vi "MAIN PS.vi"(11 "Elettrotest PS 2":refnum<vi>) -> ()   [LabVIEW 2019]
uses:
  TypeDef/ELATTROTEST PS.ctl
  TypeDef/DEVICE NAME.ctl
  <vilib>/Utility/file.llb/Read From Spreadsheet File (string).vi
  <vilib>/Instr/_visa.llb/VISA Configure Serial Port (Instr).vi
  Freq elettrotest PS global.vi
panel:
  out "error out 3":errorcluster
  out "# elements in queue":i32
  in  "Elettrotest PS":T1={"TENSIONE[V]"=230.0, "FREQ[Hz]"=50.0, "T rampa[s]"=5.0, "imposta"=FALSE, "V out [Hz]"=0.0, "F out [Hz]"=0.0, "ACK"=FALSE, "Remoto?"=FALSE, "ctrl remoto"=FALSE} {"FREQ[Hz]" min=45.0 max=65.0; "TENSIONE[V]" min=0.0 max=500.0}
  out "CK DATO":bool
  in  "remoto":bool
  in  "s":bool
  in  "SET RAMPE":bool
  in  "COMANDO":T2={"NU"=FALSE, "OUT"=FALSE, "REMOTO"=TRUE, "DC"=FALSE, "SINK"=FALSE, "MONO"=FALSE, "SENSE"=FALSE, "PORTATA"=TRUE}
  in  "rampa tensione frequenza all 2":T3
  out "Numeric":i32
  out "ACK":bool
  out "Timeout":bool
  out "Error Out":bool
  out "CK Tot":bool
  in  "EXIT":bool
  in  "Tab Control":enum32{"COM SETTINGS", "Page 2"}(tab)
  in  "baud rate (9600)":u32=1200
  in  "data bits (8)":u16=8 min=5 max=8 step=1
  in  "parity (0:none)":enum16{"None", "Odd", "Even", "Mark", "Space"}(ring)
  in  "timeout (10sec)":u32=10000
  in  "termination char\n(0xA = '\\n' = LF)":u8=10 format="%.0x"
  in  "stop bits (10: 1 bit)":u16(ring)=10 items=["1.0"=10, "1.5"=15, "2.0"=20]
  in  "Enable Termination\nChar (T)":bool=TRUE
  out "error out":errorcluster
  out "COM":string
  out "error out 2":errorcluster
  out "Fase R":T4 {"Freq" format="%#.2g"; "Vout" format="%#.1f"; "Vset" format="%#.1f"}
  out "Fase S":T4 {"Fase" format="%#.0f"; "Freq" format="%#.2g"; "Vout" format="%#.1f"; "Vset" format="%#.1f"}
  out "Fase T":T4 {"Fase" format="%#.1f"; "Freq" format="%#.2g"; "Vout" format="%#.1f"; "Vset" format="%#.1f"}
  out "Modo R":T5
  out "Modo S":T5
  out "Modo T":T5
  out "Allarme S":T6
  out "Allarme R":T6
  out "AllarmeT":T6
  in  "flow control (0:none)":u16(ring) items=["None", "XON/XOFF", "RTS/CTS", "XON/XOFF & RTS/CTS", "DTR/DSR", "XON/XOFF & DTR/DSR"]
  out "STATO":string
  in  "rampa tensione frequenza":T7 {"tiporampa" items=["Tensione"=0, "Frequenza"=1, "Fase"=3]}
  in  "rampa tensione frequenza all":T3
  # "COMANDO T\\F"
  # "INVIA COMANDO"
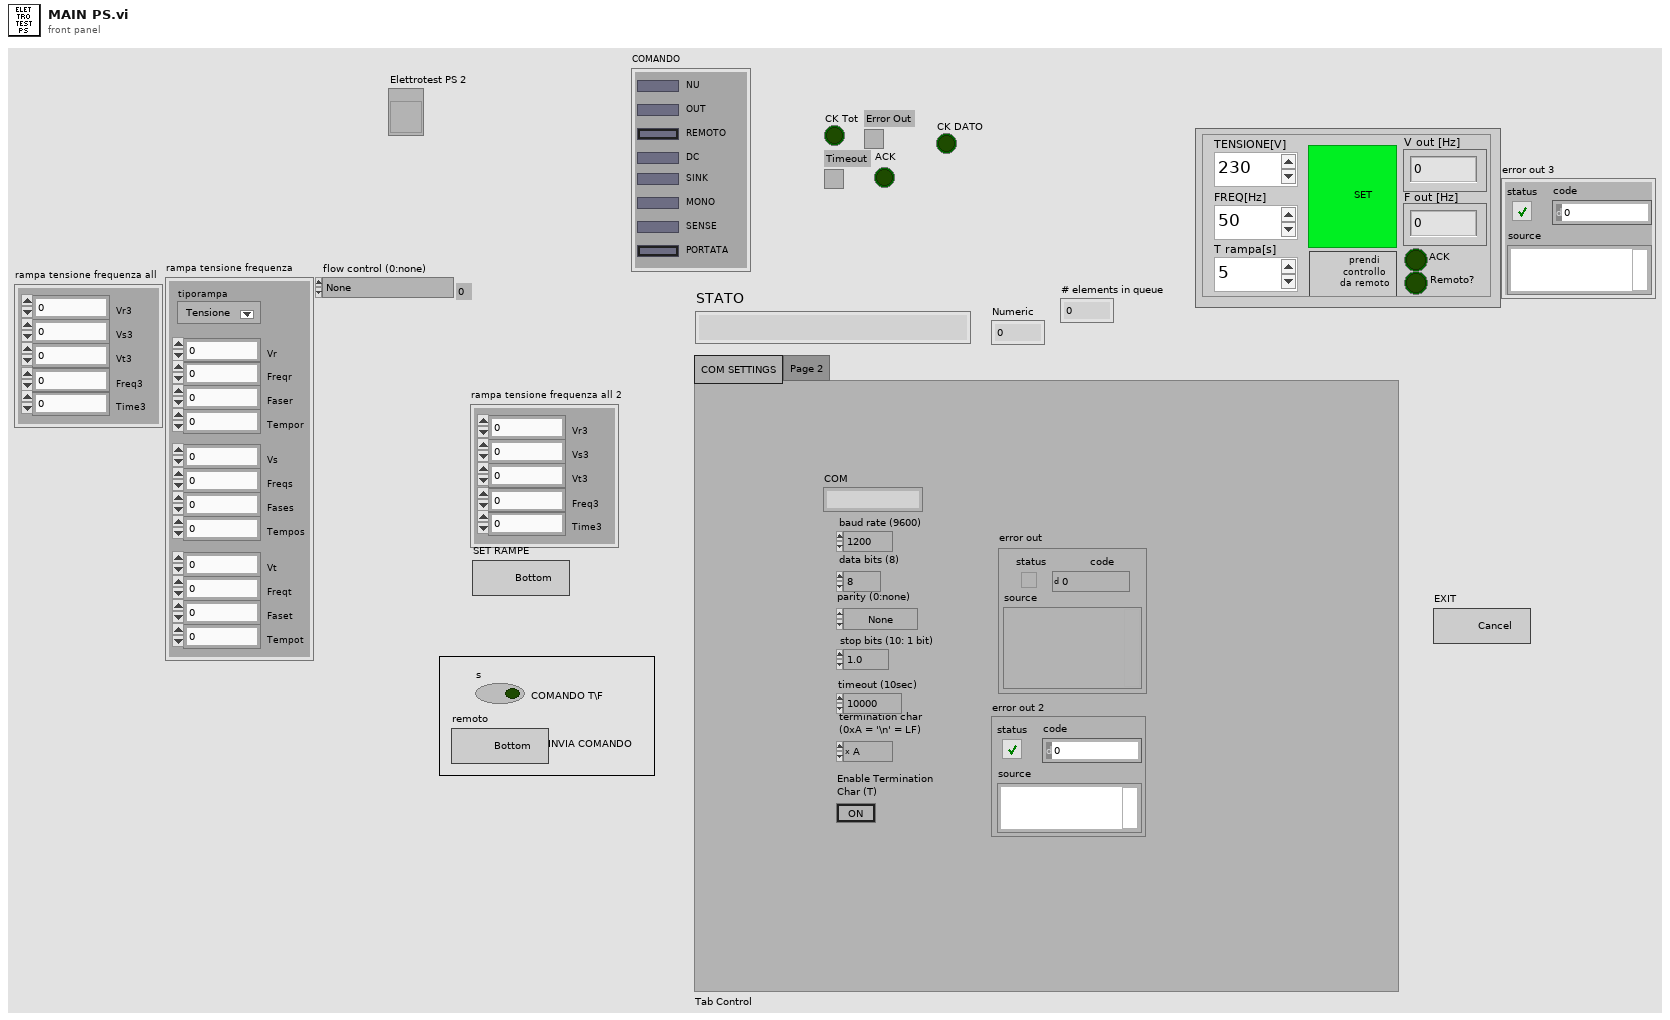
[diagram p1: front panel]
types:
  T1 = typedef "ELATTROTEST PS.ctl" = cluster{"TENSIONE[V]":dbl, "FREQ[Hz]":dbl, "T rampa[s]":dbl, "imposta":bool, "V out [Hz]":dbl, "F out [Hz]":dbl, "ACK":bool, "Remoto?":bool, "ctrl remoto":bool}
  T2 = cluster{"NU":bool, "OUT":bool, "REMOTO":bool, "DC":bool, "SINK":bool, "MONO":bool, "SENSE":bool, "PORTATA":bool}
  T3 = cluster{"Vr3":dbl, "Vs3":dbl, "Vt3":dbl, "Freq3":dbl, "Time3":dbl}
  T4 = cluster{"Vset":dbl, "Vout":dbl, "Iout":dbl, "Freq":dbl, "Fase":dbl, "Modo":dbl, "Allarmi":dbl}
  T5 = cluster{"Remote":bool, "3 Phase":bool, "DC":bool, "Portata alta":bool, "Out abilitata":bool, "Inrush abilitato":bool, "Sincronismo interno":bool, "4 Fili":bool}
  T6 = cluster{"Overvoltage":bool, "Undervoltage":bool, "Overtemperature":bool, "Inverter":bool, "Not used":bool, "DeltaV":bool, "Current limitation":bool, "Not used":bool}
  T7 = cluster{"Vr":dbl, "Tempor":dbl, "Freqr":dbl, "Faser":dbl, "Vs":dbl, "Freqs":dbl, "Fases":dbl, "Tempos":dbl, "Vt":dbl, "Freqt":dbl, "Faset":dbl, "Tempot":dbl, "tiporampa":u8}
  T8 = typedef "DEVICE NAME.ctl" = enum16{"WATTMETRO", "APLUS", "PLC BANCO 1", "PLC RACK", "PLC BANCO 2", "PS", "NI cDAQ", "RESISTOMAT"}
  T9 = enum16{"ALIGN -CENTER", "ALIGN -TOP LEFT", "ALIGN -AS IS", "ALIGN -CUSTOM"}
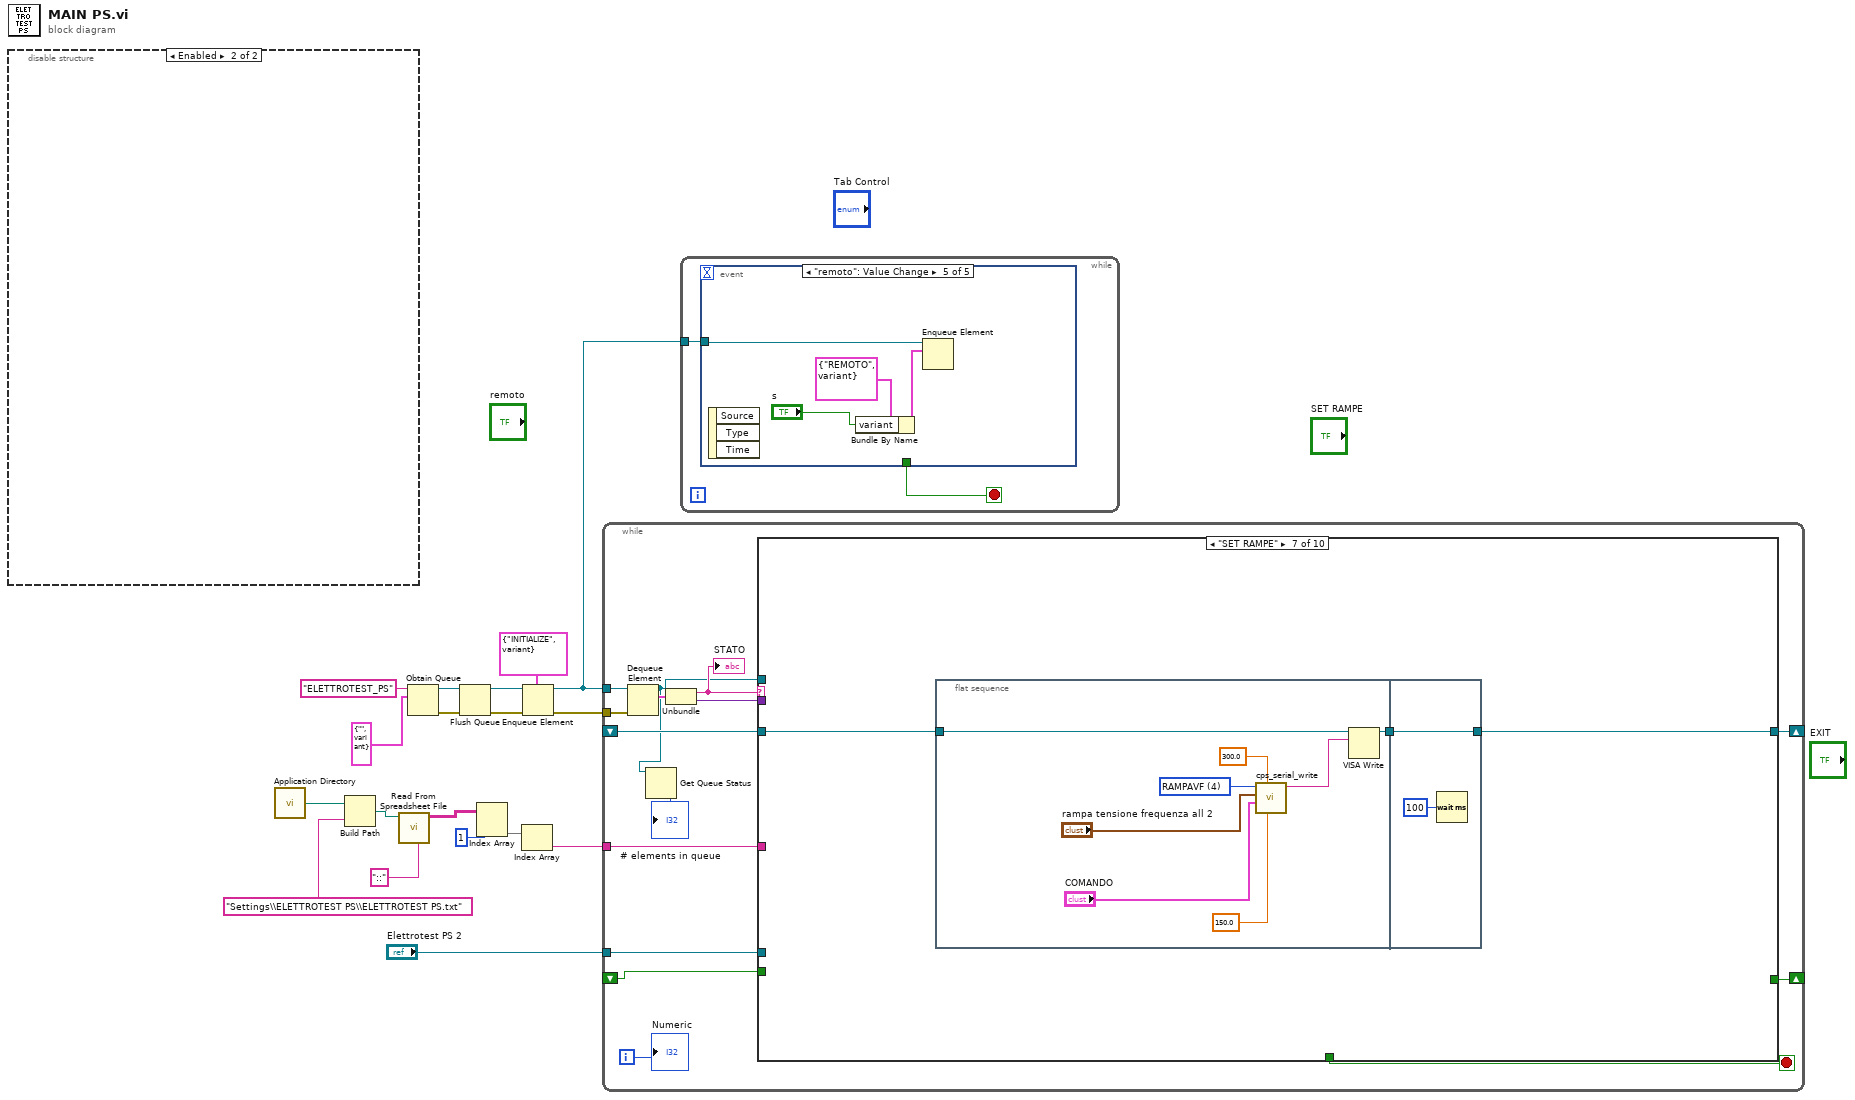
[diagram p0: block diagram]
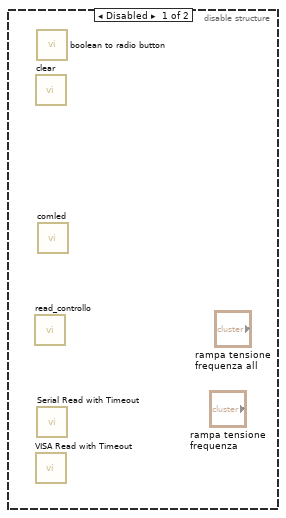
[diagram p2: hidden frame]
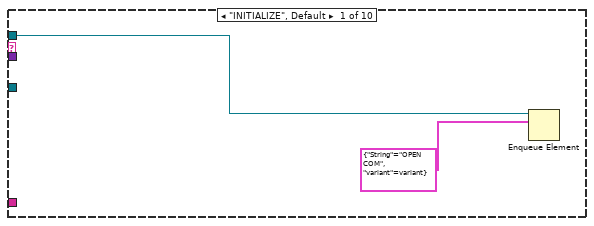
[diagram p3: hidden frame]
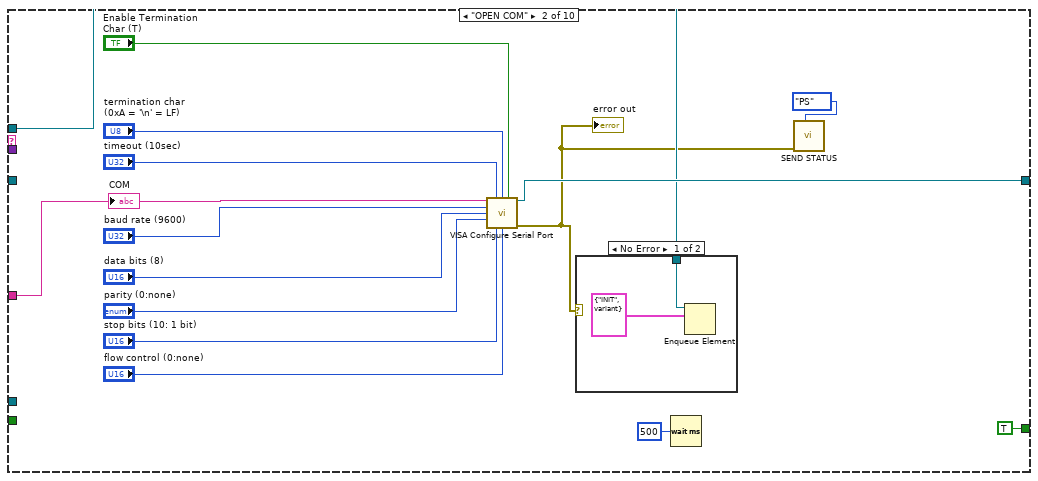
[diagram p4: hidden frame]
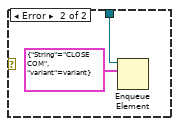
[diagram p5: hidden frame]
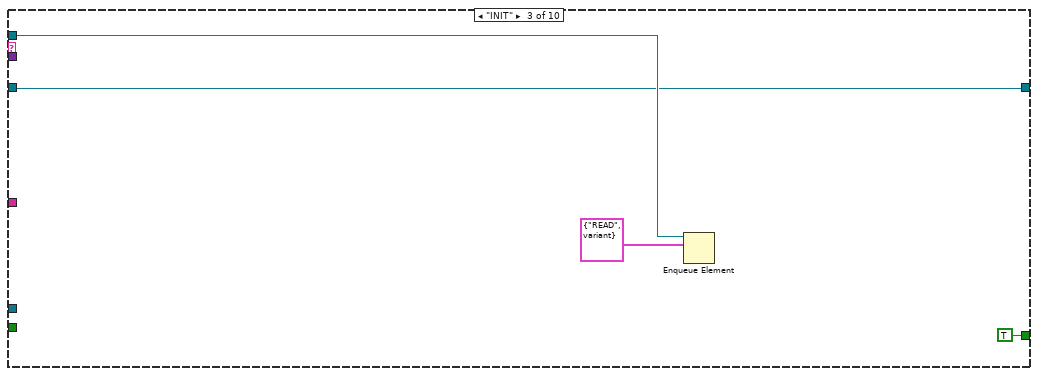
[diagram p6: hidden frame]
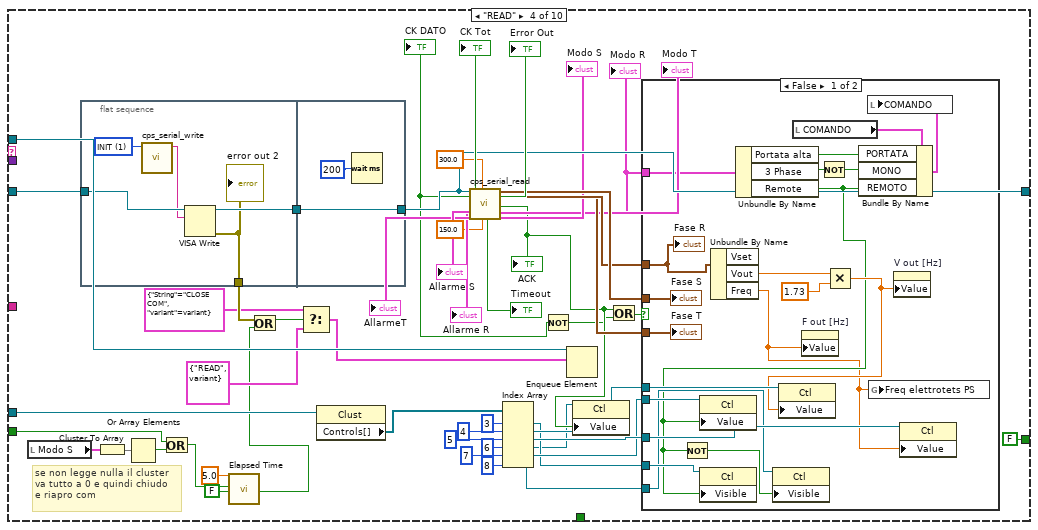
[diagram p7: hidden frame]
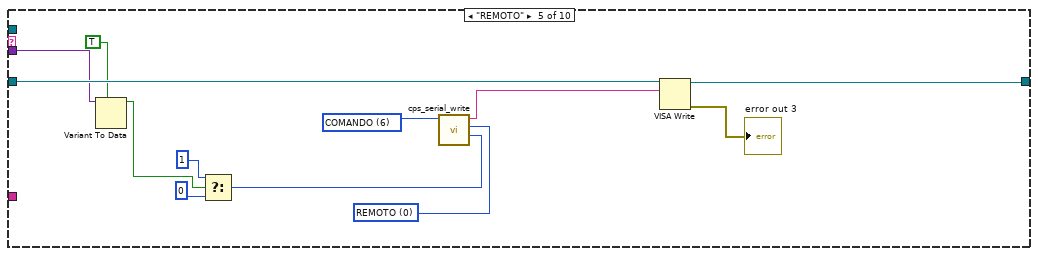
[diagram p9: hidden frame]
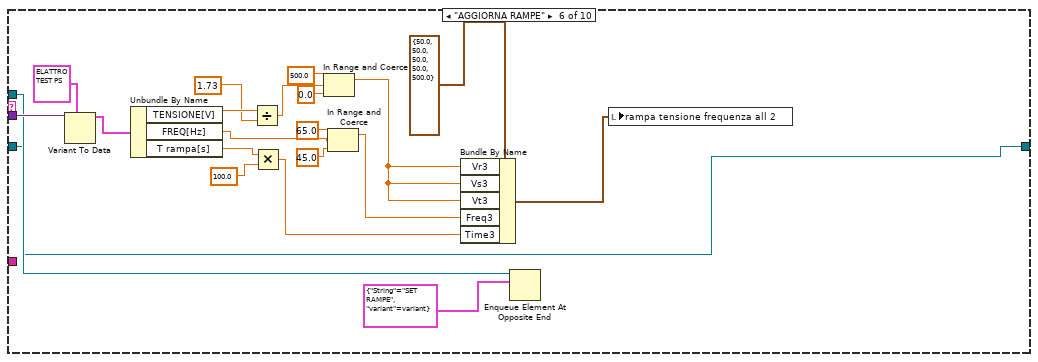
[diagram p10: hidden frame]
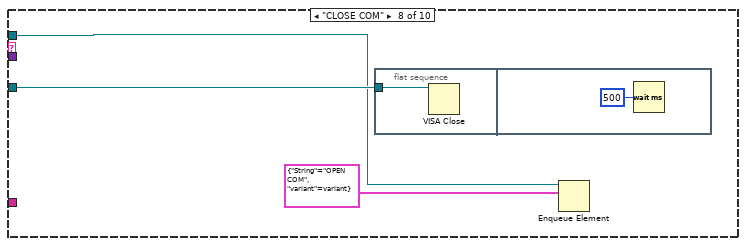
[diagram p11: hidden frame]
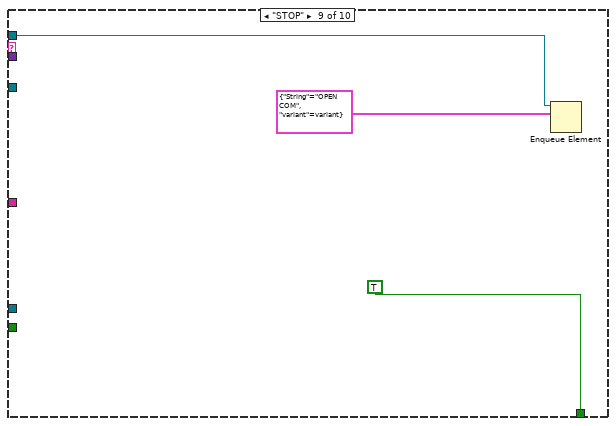
[diagram p12: hidden frame]
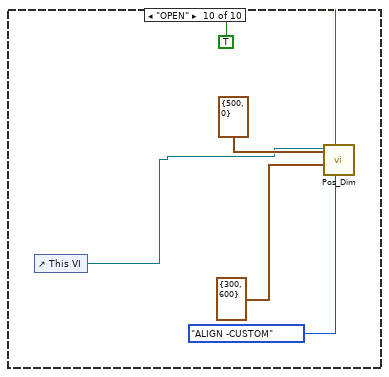
[diagram p13: hidden frame]
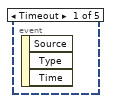
[diagram p14: hidden frame]
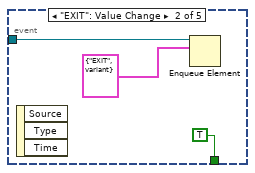
[diagram p15: hidden frame]
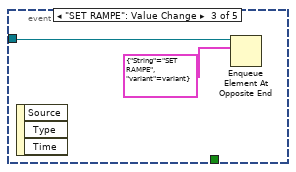
[diagram p16: hidden frame]
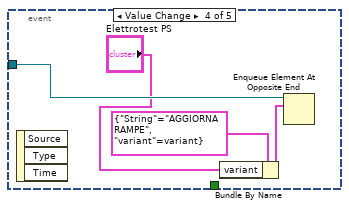
[diagram p17: hidden frame]
diagram:
  n1 = disable-structure shown="Enabled" {
    frame Disabled {
      n2 = call "read_controllo.vi"() -> ()  [unwired: 8 in, 1 out]
      n3 = call "clear.vi"() -> ()  [unwired: 1 in]
      n4 = call "VISA Read with Timeout.vi"() -> ()  [unwired: 4 in, 5 out]
      n5 = call "boolean to radio button.vi"() -> ()  [unwired: 1 in, 1 out]
      n6 = call "Serial Read with Timeout.vi"() -> ()  [unwired: 3 in, 3 out]
      n7 = call "comled.vi"() -> ()  [unwired: 1 in, 1 out]
    }
    frame Enabled {
    }
  }
  n8 = call <vilib>:"Application Directory.vi"() -> ("Application Directory"=w3:path)
  n9 = Build Path(base path=w3, name or relative path="Settings\\ELETTROTEST PS\\ELETTROTEST PS.txt") -> (appended path=w5:path)
  n10 = call-poly <vilib>:"Read From Spreadsheet File.vi"("delimiter (\\t)"="::" ("delimiter (\\t)"), "file path (dialog if empty)"=w5) -> ("all rows"=w7:string[][])  [unwired: 5 in, 4 out]
  n11 = Obtain Queue(name (unnamed)="ELETTROTEST_PS", element data type=cluster{"String":string, "variant":variant} {"String"="", "variant"=variant} ("element")) -> (queue out=w16:refnum<queue>, error out=w15:errorcluster)  [unwired: 3 in, 1 out]
  n12 = Flush Queue(queue=w16, error in (no error)=w15) -> (queue out=w14:refnum<queue>, error out=w13:errorcluster)  [unwired: 1 out]
  n13 = Index Array(array=w7, index (col)=1 ("disabled index (col)")) -> (element=w9:string[])  [unwired: 1 in]
  n14 = Index Array(array=w9) -> (element=w2:string)  [unwired: 1 in]
  n15 = Enqueue Element(queue=w14, element=cluster{"String":string, "variant":variant} {"String"="INITIALIZE", "variant"=variant}, error in (no error)=w13) -> (queue out=w10:refnum<queue>, error out=w12:errorcluster)  [unwired: 1 in, 1 out]
  n16 = while {
    tunnel: w10 -> [w33]
    tunnel: w12 -> [w32]
    shift-right: [w30] -> _
    shift-left: _ -> [w28]
    tunnel: w2 -> [w26]
    tunnel: "Elettrotest PS 2" -> [w25]
    shift-right: [w21] -> _
    shift-left: _ -> [w22]
    i -> [w27]
    stop <- w29 stop-if-true
    n17 = Dequeue Element(queue=w33, error in (no error)=w32) -> (queue out=w24:refnum<queue>, element=w35:cluster{"String":string, "variant":variant})  [unwired: 1 in, 2 out]
    n18 = Get Queue Status(queue=w24) -> (# elements in queue=→"# elements in queue":i32)  [unwired: 2 in, 7 out]
    n19 = Unbundle(w35) -> ("String"=w34:string, "variant"=w31:variant)
    "STATO" <- w34
    n20 = case shown="\"SET RAMPE\"" w34 {
      tunnel: w31 -> [_ _ _ _ w141 w170 _ _ _ _]
      tunnel: w24 -> [w37 w43 w59 w106 _ w160 _ w185 w189 _]
      tunnel: [_ w44 w58 w102 w148 w159 w172 _ _ _] -> w30
      tunnel: [_ _ _ _ _ _ _ _ TRUE _] -> w29
      tunnel: w28 -> [_ _ w58 w103 w149 w159 w173 w186 _ _]
      tunnel: w26 -> [_ w42 _ _ _ _ _ _ _ _]
      tunnel: w25 -> [_ _ _ w93 _ _ _ _ _ _]
      tunnel: w22 -> [_ _ _ w62 _ _ _ _ _ _]
      tunnel: [_ TRUE TRUE FALSE _ _ _ _ _ _] -> w21
      frame "INITIALIZE", Default {
        n21 = Enqueue Element(queue=w37, element=cluster{"String":string, "variant":variant} {"String"="OPEN COM", "variant"=variant}) -> ()  [unwired: 2 in, 3 out]
      }
      frame "OPEN COM" {
        n22 = call-poly "VISA Configure Serial Port"("VISA resource name"=w42, "timeout (10sec)"="timeout (10sec)", "termination char\n(0xA = '\\n' = LF)"="termination char\n(0xA = '\\n' = LF)", "Enable Termination\nChar (T)"="Enable Termination\nChar (T)", "baud rate (9600)"="baud rate (9600)", "data bits (8)"="data bits (8)", "parity (0:none)"="parity (0:none)", "stop bits (10: 1 bit)"="stop bits (10: 1 bit)", "flow control (0:none)"="flow control (0:none)") -> ("VISA resource name out"=w44:refnum<visa-resource-name>, "error out"=w39:errorcluster)  [unwired: 5 in]
        "error out" <- w39
        n23 = case shown="No Error" w39 {
          tunnel: w43 -> [w53 w55]
          frame No Error {
            n24 = Enqueue Element(queue=w53, element=cluster{"String":string, "variant":variant} {"String"="INIT", "variant"=variant}) -> ()  [unwired: 2 in, 3 out]
          }
          frame Error {
            n25 = Enqueue Element(queue=w55, element=cluster{"String":string, "variant":variant} {"String"="CLOSE COM", "variant"=variant}) -> ()  [unwired: 2 in, 3 out]
          }
        }
        n26 = Wait (ms)(milliseconds to wait=u32 500) -> ()  [unwired: 1 out]
        n27 = call "SEND STATUS.vi"("ELEMENT"=DEVICE_NAME."PS", "error in (no error)"=w39) -> ()  [unwired: 9 in, 1 out]
        "COM" <- w42
      }
      frame "INIT" {
        n28 = Enqueue Element(queue=w59, element=cluster{"String":string, "variant":variant} {"String"="READ", "variant"=variant}) -> ()  [unwired: 2 in, 3 out]
      }
      frame "READ" {
        # "se non legge nulla il cluster\nva tutto a 0 e quindi chiudo\ne riapro com"
        n29 = local read "Modo S"() -> (w78:T5)
        n30 = flat-sequence {
          tunnel: w103 -> [w135]
          tunnel: [w134] -> w99
          tunnel: [w131] -> w89
          tunnel: [w137] -> w102
          tunnel: w99 -> [w137]
          frame #0 {
            w133 = u8 1 items=["NONE", "INIT", "ACQ", "SETMD", "RAMPAVF", "RAMPAPAR", "COMANDO"] ("CODE")
            n31 = call "cps_serial_write.vi"("CODE"=w133) -> ("Pacchetto"=w132:string)  [unwired: 8 in]
            n32 = VISA Write(VISA resource name=w135, write buffer=w132) -> (VISA resource name out=w134:refnum<visa-resource-name>, error out=w131:errorcluster)  [unwired: 1 in, 1 out]
            "error out 2" <- w131
          }
          frame #1 {
            n33 = Wait (ms)(milliseconds to wait=u32 200) -> ()  [unwired: 1 out]
          }
        }
        n34 = Cluster To Array(cluster=w78) -> (array=w77:bool[])
        n35 = Or Array Elements(Boolean array=w77) -> (logical OR=w75:bool)
        n36 = Or(x=w62, y=w75) -> (x .or. y?=w63:bool)
        n37 = call "Elapsed Time"("Time Target (s)"=5.0, "Reset"=w63, "Auto Reset"=FALSE) -> ("Time has Elapsed"=w73:bool)  [unwired: 9 in, 7 out]
        n38 = Or(x=w89, y=w73) -> (x .or. y?=w76:bool)
        n39 = Select(t=cluster{"String":string, "variant":variant} {"String"="CLOSE COM", "variant"=variant} ("element"), s=w76, f=cluster{"String":string, "variant":variant} {"String"="READ", "variant"=variant} ("element")) -> (s? t:f=w86:cluster{"String":string, "variant":variant})
        n40 = property class="Clust"(reference=w93) -> ("Controls[]"=w71:refnum<vi>[])  [unwired: 1 in, 2 out]
        n41 = call "cps_serial_read.vi"("serial in"=w102, "Range H"=300.0, "Range L"=150.0) -> ("CK DATO"=w81:bool, "Allarme S"=→"Allarme S":T6, "AllarmeT"=→"AllarmeT":T6, "CK Tot"=→"CK Tot":bool, "Allarme R"=→"Allarme R":T6, "Error Out"=→"Error Out":bool, "Timeout"=→"Timeout":bool, "Fase R"=w105:T4, "Modo T"=→"Modo T":T5, "Fase S"=w107:T4, "Fase T"=w104:T4, "ACK"=w90:bool, "Modo R"=w79:T5, "Modo S"=→"Modo S":T5)  [unwired: 1 in, 2 out]
        "ACK" <- w90
        "Modo R" <- w79
        "CK DATO" <- w81
        n42 = Index Array(array=w71, index #1=3 ("index"), index #2=4 ("index"), index #3=5 ("index"), index #4=6 ("index"), index #5=7 ("index"), index #6=8 ("index")) -> (element #1=w84:refnum<vi>, element #2=w92:refnum<vi>, element #3=w91:refnum<vi>, element #4=w68:refnum<vi>, element #5=w85:refnum<vi>, element #6=w83:refnum<vi>)
        n43 = Not(x=w81) -> (.not. x?=w80:bool)
        n44 = Enqueue Element(queue=w106, element=w86) -> ()  [unwired: 2 in, 3 out]
        n45 = property class="Ctl"(reference=w68, "Value"=w90) -> ()  [unwired: 1 in, 2 out]
        n46 = Or(x=w90, y=w80) -> (x .or. y?=w82:bool)
        n47 = case shown="False" w82 {
          tunnel: w107 -> [w130 _]
          tunnel: w105 -> [w125 _]
          tunnel: w104 -> [w129 _]
          tunnel: w92 -> [w128 _]
          tunnel: w91 -> [w127 _]
          tunnel: w85 -> [w126 _]
          tunnel: w84 -> [w124 _]
          tunnel: w83 -> [w123 _]
          tunnel: w79 -> [w122 _]
          frame False {
            n48 = Unbundle By Name(w125) -> ("Vout"=w121:dbl, "Freq"=w111:dbl)  [unwired: 1 out]
            n49 = Unbundle By Name(w122) -> ("Portata alta"=w115:bool, "3 Phase"=w114:bool, "Remote"=w112:bool)
            n50 = Not(x=w112) -> (.not. x?=w118:bool)
            n51 = property class="Ctl"(reference=w126, "Value"=w112) -> ()  [unwired: 1 in, 2 out]
            n52 = property class="Ctl"(reference=w124, "Visible"=w112) -> ()  [unwired: 1 in, 2 out]
            n53 = property class="Ctl"(reference=w123, "Visible"=w118) -> ()  [unwired: 1 in, 2 out]
            n54 = local read "COMANDO"() -> (w116:T2)
            n55 = property on="F out [Hz]" class="DigNum (strict)"("Value"=w111) -> ()  [unwired: 2 in, 2 out]
            n56 = Not(x=w114) -> (.not. x?=w113:bool)
            n57 = Multiply(x=w121, y=1.73) -> (x*y=w119:dbl)
            n58 = property class="Ctl"(reference=w128, "Value"=w119) -> ()  [unwired: 1 in, 2 out]
            n59 = Bundle By Name(cluster=w116, "PORTATA"=w115, "MONO"=w113, "REMOTO"=w112) -> (w117:T2)
            n60 = local write "COMANDO"(w117) -> ()
            n61 = global write "Freq elettrotest PS global.vi" "Freq elettrotets PS"(w111) -> ()
            n62 = property on="V out [Hz]" class="DigNum (strict)"("Value"=w119) -> ()  [unwired: 2 in, 2 out]
            n63 = property class="Ctl"(reference=w127, "Value"=w111) -> ()  [unwired: 1 in, 2 out]
            "Fase S" <- w130
            "Fase R" <- w125
            "Fase T" <- w129
          }
          frame True {
          }
        }
      }
      frame "REMOTO" {
        w142 = u8 6 items=["NONE", "INIT", "ACQ", "SETMD", "RAMPAVF", "RAMPAPAR", "COMANDO"] ("CODE")
        w147 = u16 0 items=["REMOTO", "OUT", "RANGE", "SENSE", "MONO", "SINC", "DC", "INRUSH", "WAVEFORM"] ("Type (COM)")
        n64 = Variant To Data(type=TRUE, Variant=w141) -> (data=w139:bool)  [unwired: 1 in, 1 out]
        n65 = Select(t=u16 1 ("Data (COM)"), s=w139, f=u16 0) -> (s? t:f=w143:u16)
        n66 = call "cps_serial_write.vi"("Data (COM)"=w143, "Type (COM)"=w147, "CODE"=w142) -> ("Pacchetto"=w146:string)  [unwired: 6 in]
        n67 = VISA Write(VISA resource name=w149, write buffer=w146) -> (VISA resource name out=w148:refnum<visa-resource-name>, error out=→"error out 3":errorcluster)  [unwired: 1 in, 1 out]
      }
      frame "AGGIORNA RAMPE" {
        n68 = Variant To Data(type=T1 {"TENSIONE[V]"=230.0, "FREQ[Hz]"=50.0, "T rampa[s]"=5.0, "imposta"=FALSE, "V out [Hz]"=50.30307692307692, "F out [Hz]"=50.0, "ACK"=FALSE, "Remoto?"=FALSE, "ctrl remoto"=FALSE} ("Elettrotest PS"), Variant=w170) -> (data=w169:T1)  [unwired: 1 in, 1 out]
        n69 = Unbundle By Name(w169) -> ("TENSIONE[V]"=w168:dbl, "FREQ[Hz]"=w152:dbl, "T rampa[s]"=w166:dbl)
        n70 = Divide(x=w168, y=1.73) -> (x/y=w158:dbl)
        n71 = Multiply(x=w166, y=100.0) -> (x*y=w163:dbl)
        n72 = In Range and Coerce(upper limit=500.0, x=w158, lower limit=0.0) -> (coerced(x)=w155:dbl)  [unwired: 1 out]
        n73 = In Range and Coerce(upper limit=65.0, x=w152, lower limit=45.0) -> (coerced(x)=w151:dbl)  [unwired: 1 out]
        n74 = Bundle By Name(cluster=T3 {"Vr3"=50.0, "Vs3"=50.0, "Vt3"=50.0, "Freq3"=50.0, "Time3"=500.0} ("rampa tensione frequenza all 2"), "Vr3"=w155, "Vs3"=w155, "Vt3"=w155, "Freq3"=w151, "Time3"=w163) -> (w162:T3)
        n75 = Enqueue Element At Opposite End(queue=w160, element=cluster{"String":string, "variant":variant} {"String"="SET RAMPE", "variant"=variant}) -> ()  [unwired: 2 in, 3 out]
        n76 = local write "rampa tensione frequenza all 2"(w162) -> ()
      }
      frame "SET RAMPE" {
        n77 = flat-sequence {
          tunnel: [w177] -> w171
          tunnel: w173 -> [w178]
          tunnel: [w183] -> w172
          tunnel: w171 -> [w183]
          frame #0 {
            w179 = u8 4 items=["NONE", "INIT", "ACQ", "SETMD", "RAMPAVF", "RAMPAPAR", "COMANDO"] ("CODE")
            n78 = call "cps_serial_write.vi"("Range L"=150.0, "Range H"=300.0, "COMANDO"="COMANDO", "rampa tensione frequenza all"="rampa tensione frequenza all 2", "CODE"=w179) -> ("Pacchetto"=w176:string)  [unwired: 4 in]
            n79 = VISA Write(VISA resource name=w178, write buffer=w176) -> (VISA resource name out=w177:refnum<visa-resource-name>)  [unwired: 1 in, 2 out]
          }
          frame #1 {
            n80 = Wait (ms)(milliseconds to wait=u32 100) -> ()  [unwired: 1 out]
          }
        }
      }
      frame "CLOSE COM" {
        n81 = flat-sequence {
          tunnel: w186 -> [w187]
          frame #0 {
            n82 = VISA Close(VISA resource name=w187) -> ()  [unwired: 1 in, 1 out]
          }
          frame #1 {
            n83 = Wait (ms)(milliseconds to wait=u32 500) -> ()  [unwired: 1 out]
          }
        }
        n84 = Enqueue Element(queue=w185, element=cluster{"String":string, "variant":variant} {"String"="OPEN COM", "variant"=variant}) -> ()  [unwired: 2 in, 3 out]
      }
      frame "STOP" {
        n85 = Enqueue Element(queue=w189, element=cluster{"String":string, "variant":variant} {"String"="OPEN COM", "variant"=variant}) -> ()  [unwired: 2 in, 3 out]
      }
      frame "OPEN" {
        n86 = control-ref of="This VI"() -> (w192:refnum<vi>)
        n87 = call "Pos_Dim.vi"("Mode"=T9."ALIGN -CUSTOM", "Open FP"=TRUE, "Size"=cluster{"right":i16, "bottom":i16} {"right"=300, "bottom"=600}, "Poistion"=cluster{"left":i16, "top":i16} {"left"=500, "top"=0}, "VIRefNum  IN"=w192) -> ()  [unwired: 2 in, 5 out]
      }
    }
    "Numeric" <- w27
  }
  n88 = while {
    tunnel: w10 -> [w197]
    stop <- w198 stop-if-true
    n89 = event shown="[4] \"remoto\": Value Change" {
      selector: _ -> [_ _ _ _ _]
      dyn-events: _ -> [_ _ _ _ _]
      timeout: _ -> [_ _ _ _ _]
      tunnel: [_ TRUE _ _ _] -> w198
      tunnel: w197 -> [_ w200 w202 w207 w211]
      event Timeout {
        n90 = event-data() -> ()  [unwired: 1 in, 3 out]
      }
      event "EXIT": Value Change {
        n91 = event-data() -> ()  [unwired: 1 in, 3 out]
        n92 = Enqueue Element(queue=w200, element=cluster{"String":string, "variant":variant} {"String"="EXIT", "variant"=variant}) -> ()  [unwired: 2 in, 3 out]
      }
      event "SET RAMPE": Value Change {
        n93 = event-data() -> ()  [unwired: 1 in, 3 out]
        n94 = Enqueue Element At Opposite End(queue=w202, element=cluster{"String":string, "variant":variant} {"String"="SET RAMPE", "variant"=variant}) -> ()  [unwired: 2 in, 3 out]
      }
      event Value Change {
        n95 = event-data() -> ()  [unwired: 1 in, 3 out]
        n96 = Bundle By Name(cluster=cluster{"String":string, "variant":variant} {"String"="AGGIORNA RAMPE", "variant"=variant} ("element"), "variant"="Elettrotest PS") -> (w205:cluster{"String":string, "variant":variant})
        n97 = Enqueue Element At Opposite End(queue=w207, element=w205) -> ()  [unwired: 2 in, 3 out]
      }
      event "remoto": Value Change {
        n98 = event-data() -> ()  [unwired: 1 in, 3 out]
        n99 = Bundle By Name(cluster=cluster{"String":string, "variant":variant} {"String"="REMOTO", "variant"=variant} ("element"), "variant"="s") -> (w208:cluster{"String":string, "variant":variant})
        n100 = Enqueue Element(queue=w211, element=w208) -> ()  [unwired: 2 in, 3 out]
      }
    }
  }
